vi "Test_Putty_PXI.vi"(4 "error in":errorcluster, 7 "Parameter Array in":string[](array[string])) -> (0 "error out":errorcluster, 1 "Result Paragraphs":string[](array[string]), 2 "Pass":bool, 3 "Parameter Array Out":string[](array[string]))   [LabVIEW 2018]
uses:
  CommonSubVIs/Framework/Flattened_Array/Test Parameter Enum.ctl
  CommonSubVIs/Framework/Flattened_Array/Get Parameter Value by Name (String).vi
panel:
  in  "Tab Control":enum32{"Connector Pane controls", "The rest"}(tab)
  in  "Network Address":string="10.0.62.162"
  in  "operation (0:open)":T1(ring)
  in  "Cammand need to be Executed":string
  out "Value":string
  in  "Putty location":string="C:\\Users\\nitest\\Desktop\\putty[32bit].exe "
  in  "Username":string="lvadmin"
  in  "Host name /ip":string="10.0.86.122"
  in  "Operation":string=" -ssh"
  in  "-pw":string=" -pw"
  in  "Password":string=" labview==="
  in  "-m":string=" -m "
  # "This VI is used to run cammands\n from Linux Dev machine"
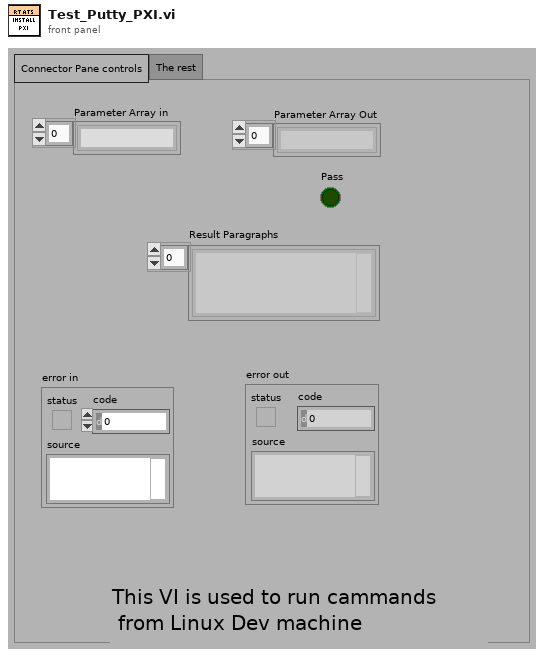
[diagram p1: front panel]
types:
  T1 = enum16{"open", "replace", "create", "open or create", "replace or create", "replace or create with confirmation"}
  T2 = typedef "Test Parameter Enum.ctl" = enum16{"Main Test Target IP", "Main Test Target Name", "Main Test Target Alias", "Main Host IP", "Default Target Alias", "Default Target Host Name", "Dafault Target IP Address", "Dafault Target LV Date", "Available Targets", "Target Alias by Index", "Target IP by Alias", "Target IP by  Index", "Current Iteration", "Total Iterations", "Test Project Name", "Current Test Result", "Current Test Name", "Current Test Logical Path", "Test Folder", "Configuration Name", "Configuration Index", "Total Configurations", "Performance Values", "Result Paragraphs", "Connector Pane", "Avoid?", "Avoid Reason", "Case Name", "Case #", "Total Cases", "Case Data", "Disable reason"}
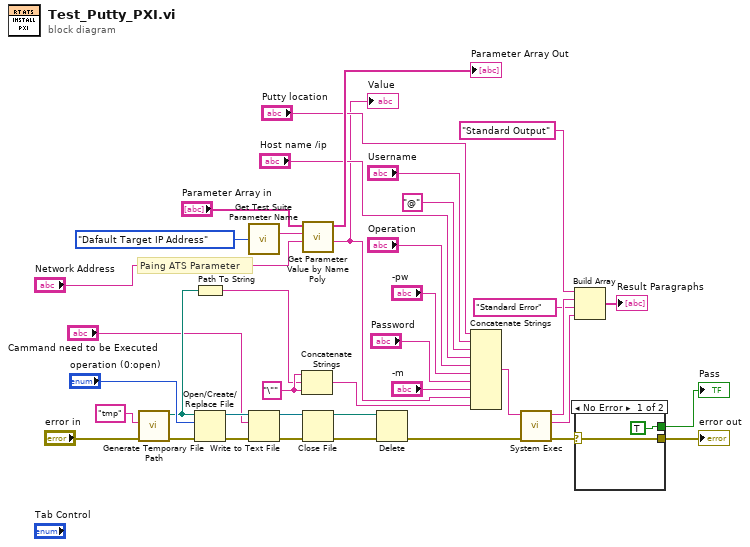
[diagram p0: block diagram]
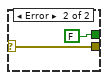
[diagram p2: hidden frame]
diagram:
  w6 = "\"" ("string")
  # "Paing ATS Parameter"
  n1 = call <vilib>:"Generate Temporary File Path.vi"("error in (no error)"="error in", "Temporary File Extension (tmp)"="tmp") -> ("error out"=w33:errorcluster, "Unique Temporary File Path"=w7:path)  [unwired: 8 in]
  n2 = Path To String(path=w7) -> (string=w5:string)
  n3 = Open/Create/Replace File(file path (use dialog)=w7, error in=w33, operation (0:open)="operation (0:open)") -> (refnum out=w30:refnum<file>, error out=w31:errorcluster)  [unwired: 3 in, 1 out]
  n4 = call "Get Test Suite Parameter Name.vi"("Test Suite Parameter"=Test_Parameter_Enum."Dafault Target IP Address") -> ("Parameter Name"=w36:string)  [unwired: 13 in, 1 out]
  n5 = Write to Text File(file (use dialog)=w30, text="Cammand need to be Executed", error in=w31) -> (refnum out=w24:refnum<file>, error out=w28:errorcluster)  [unwired: 1 in, 1 out]
  n6 = Concatenate Strings(w6, w5, w6) -> (w2:string)
  n7 = call-poly "Get Parameter Value by Name Poly.vi"("Default Value"="Network Address", "Parameter"=w36, "Parameter Array in"="Parameter Array in") -> ("Value"=w1:string, "Parameter Array Out"=→"Parameter Array Out":string[])  [unwired: 5 in, 1 out]
  "Value" <- w1
  n8 = Close File(refnum=w24, error in=w28) -> (path=w23:path, error out=w29:errorcluster)
  n9 = Delete(path (use dialog)=w23, error in=w29) -> (error out=w26:errorcluster)  [unwired: 3 in, 2 out]
  n10 = Concatenate Strings("Putty location", "Username", "@" ("string 3"), "Host name /ip", "Operation", "-pw", "Password", "-m", w1, w2) -> (w8:string)
  n11 = call <vilib>:"System Exec.vi"("error in (no error)"=w26, "command line"=w8) -> ("error out"=w27:errorcluster, "standard error"=w20:string, "standard output"=w21:string)  [unwired: 6 in, 1 out]
  n12 = Build Array("Standard Output" ("element"), w21, "Standard Error" ("element"), w20) -> (→"Result Paragraphs":string[])
  n13 = case shown="No Error" w27 {
    selector: w27 -> [w41 w42]
    tunnel: [TRUE FALSE] -> w39
    tunnel: [w41 w42] -> w25
    frame No Error {
    }
    frame Error {
    }
  }
  "error out" <- w25
  "Pass" <- w39
